vi "send_currentRamp-v02.vi"(0 "daq_ao":tag="Dev1/ao1", 1 "daq_ai":tag="Dev1/ai0:1", 5 "VoltageRampValuesCluster":T2, 7 "Sample Freq (Hz)":dbl min=0.0 max=40000.0, 9 "set holding (mV)":dbl, 13 "Number of Replicates":i16=1 min=1 max=10, 14 "error in":errorcluster) -> (4 "output cluster":T1, 6 "output waveform":waveform(dbl)[](graph), 8 "protocol response":waveform(dbl)[](graph) caption="jumptestMonitor", 10 "error out":errorcluster)   [LabVIEW 2019]
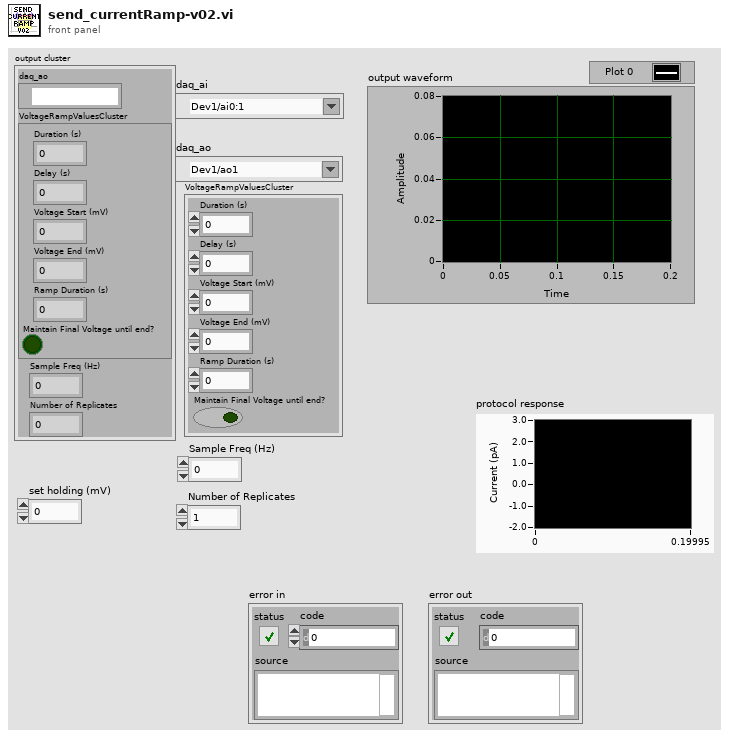
[diagram p1: front panel]
types:
  T1 = cluster{"daq_ao":tag, "VoltageRampValuesCluster":cluster{"Duration (s)":dbl, "Delay (s)":dbl, "Voltage Start (mV)":dbl, "Voltage End (mV)":dbl, "Ramp Duration (s)":dbl, "Maintain Final Voltage until end?":bool}, "Sample Freq (Hz)":dbl, "Number of Replicates":i16}
  T2 = cluster{"Duration (s)":dbl, "Delay (s)":dbl, "Voltage Start (mV)":dbl, "Voltage End (mV)":dbl, "Ramp Duration (s)":dbl, "Maintain Final Voltage until end?":bool}
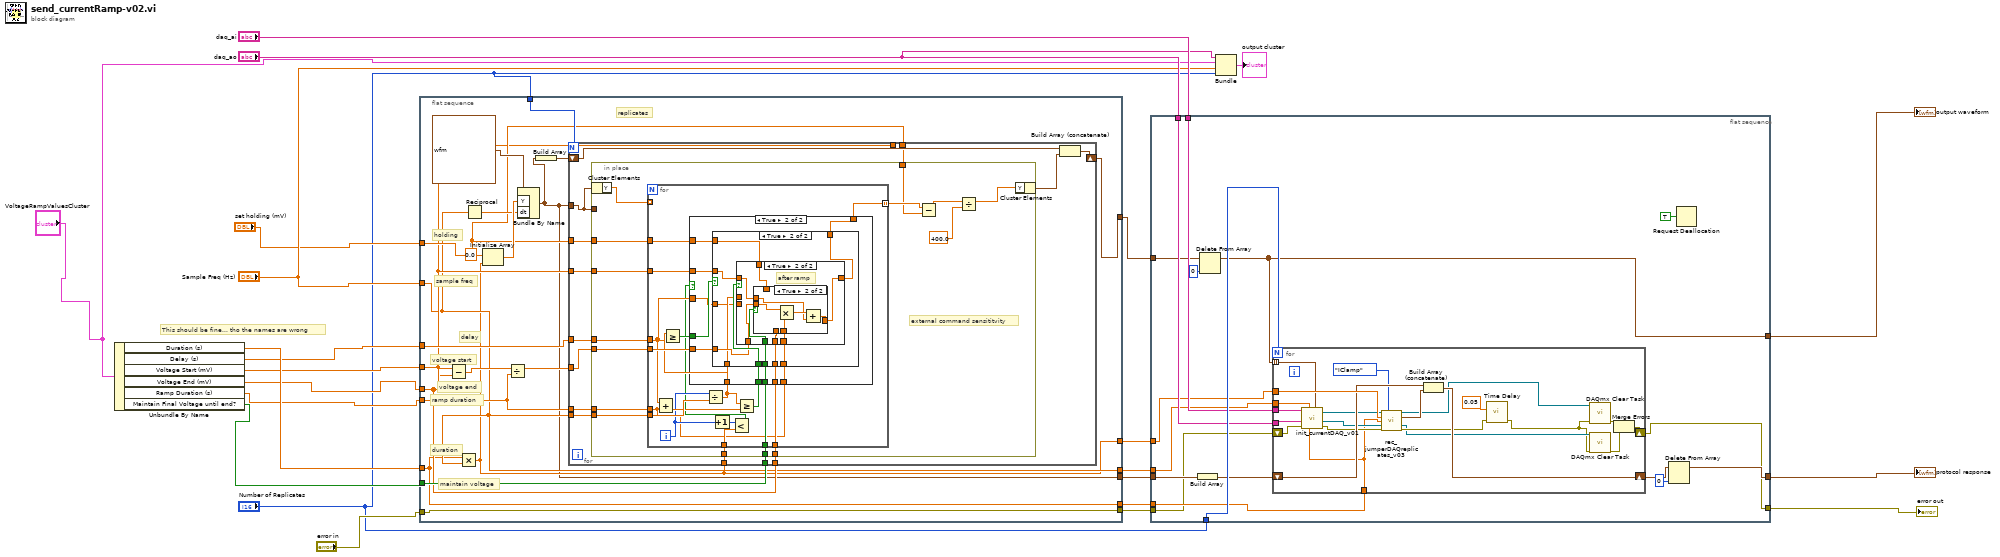
[diagram p0: block diagram]
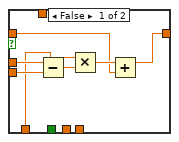
[diagram p4: hidden frame]
diagram:
  # "This should be fine... tho the names are wrong"
  n1 = Unbundle By Name("VoltageRampValuesCluster") -> ("Duration (s)"=w13:dbl, "Delay (s)"=w9:dbl, "Voltage Start (mV)"=w10:dbl, "Voltage End (mV)"=w11:dbl, "Ramp Duration (s)"=w12:dbl, "Maintain Final Voltage until end?"=w14:bool)
  n2 = flat-sequence {
    tunnel: w13 -> [w24]
    tunnel: "error in" -> [w33]
    tunnel: w9 -> [w38]
    tunnel: w10 -> [w28]
    tunnel: "Number of Replicates" -> [w43]
    tunnel: "Sample Freq (Hz)" -> [w27]
    tunnel: "set holding (mV)" -> [w30]
    tunnel: w11 -> [w31]
    tunnel: w12 -> [w37]
    tunnel: w14 -> [w35]
    tunnel: [w34] -> w5
    tunnel: [w28] -> _
    tunnel: [w33] -> w16
    tunnel: [w27] -> w4
    tunnel: [w26] -> w3
    tunnel: [w25] -> w2
    tunnel: [w24] -> w1
    frame #0 {
      # "maintain voltage"
      # "duration"
      # "ramp duration"
      # "voltage end"
      # "voltage start"
      # "delay"
      # "replicates"
      # "sample freq"
      # "holding"
      n3 = Subtract(x=w31, y=w28) -> (x-y=w32:dbl)
      n4 = Multiply(x=w24, y=w27) -> (x*y=w26:dbl)
      n5 = Reciprocal(x=w27) -> (1/x=w36:dbl)
      n6 = Initialize Array(0.0 ("element"), w26) -> (w40:dbl[])
      n7 = Divide(x=w32, y=w37) -> (x/y=w39:dbl)
      n8 = Bundle By Name(cluster=waveform(dbl) {"t0"=timestamp(0 s since 1904-01-01), "dt"=1.0, "Y"=[]} ("signal out"), "Y"=w40, "dt"=w36) -> (w25:waveform(dbl))
      n9 = Build Array(w25) -> (w42:waveform(dbl)[])
      n10 = for {
        N: w43 -> [_]
        shift-right: [w57] -> w34
        shift-left: w42 -> [w56]
        tunnel: w25 -> [w45]
        tunnel: w39 -> [w51]
        tunnel: w27 -> [w55]
        tunnel: w38 -> [w54]
        tunnel: w37 -> [w53]
        tunnel: w28 -> [w52]
        tunnel: w26 -> [w50]
        tunnel: w30 -> [w46]
        tunnel: w35 -> [w49]
        tunnel: w28 -> [_]
        tunnel: w30 -> [w48]
        tunnel: w31 -> [w47]
        n11 = in-place {
          in-place-border: w45 -> [_]
          in-place-border: w55 -> [w72]
          in-place-border: w54 -> [w71]
          in-place-border: w53 -> [w70]
          in-place-border: w52 -> [w69]
          in-place-border: w51 -> [w68]
          in-place-border: w50 -> [w67]
          in-place-border: w49 -> [w66]
          in-place-border: w48 -> [w65]
          in-place-border: w47 -> [w64]
          in-place-border: w46 -> [w61]
          # "external command sensititvity"
          n12 = in-place-cluster #1(w45) -> ("Y"=w59:dbl[])
          n13 = for {
            tunnel: [w73] -> w62 mode=indexing
            tunnel: w72 -> [w89]
            tunnel: w71 -> [w82]
            tunnel: w70 -> [w74]
            tunnel: w69 -> [w86]
            tunnel: w68 -> [w85]
            tunnel: w67 -> [w81]
            tunnel: w66 -> [w77]
            tunnel: w65 -> [w76]
            tunnel: w64 -> [w75]
            tunnel: w59 -> [_] mode=indexing
            i -> [w80]
            n14 = Add(x=w82, y=w74) -> (x+y=w83:dbl)
            n15 = Divide(x=w80, y=w89) -> (x/y=w84:dbl)
            n16 = Greater Or Equal?(x=w84, y=w82) -> (x >= y?=w88:bool)
            n17 = Increment(x=w80) -> (x+1=w78:i32)
            n18 = Less?(x=w78, y=w81) -> (x < y?=w79:bool)
            n19 = Greater Or Equal?(x=w84, y=w83) -> (x >= y?=w87:bool)
            n20 = case shown="True" w79 {
              tunnel: w88 -> [_ w101]
              tunnel: [w90 w100] -> w73
              tunnel: w87 -> [_ w99]
              tunnel: w86 -> [w90 w98]
              tunnel: w85 -> [_ w97]
              tunnel: w84 -> [_ w96]
              tunnel: w82 -> [_ w95]
              tunnel: w77 -> [_ w94]
              tunnel: w76 -> [_ w93]
              tunnel: w75 -> [_ w92]
              tunnel: w74 -> [_ w91]
              frame False {
                # "last sample"
              }
              frame True {
                n21 = case shown="True" w101 {
                  tunnel: [w102 w110] -> w100
                  tunnel: w99 -> [_ w112]
                  tunnel: w98 -> [w102 w111]
                  tunnel: w97 -> [_ w109]
                  tunnel: w96 -> [_ w108]
                  tunnel: w95 -> [_ w107]
                  tunnel: w94 -> [_ w106]
                  tunnel: w93 -> [_ w105]
                  tunnel: w92 -> [_ w104]
                  tunnel: w91 -> [_ w103]
                  frame False {
                    # "before delay"
                  }
                  frame True {
                    n22 = case shown="True" w112 {
                      tunnel: w111 -> [w113 w125]
                      tunnel: [w114 w124] -> w110
                      tunnel: w109 -> [w115 w121]
                      tunnel: w108 -> [w118 _]
                      tunnel: w107 -> [w119 _]
                      tunnel: w106 -> [_ w126]
                      tunnel: w105 -> [_ w123]
                      tunnel: w104 -> [_ w122]
                      tunnel: w103 -> [_ w120]
                      frame False {
                        n23 = Subtract(x=w118, y=w119) -> (x-y=w117:dbl)
                        n24 = Multiply(x=w115, y=w117) -> (x*y=w116:dbl)
                        n25 = Add(x=w116, y=w113) -> (x+y=w114:dbl)
                      }
                      frame True {
                        # "after ramp"
                        n26 = case shown="True" w126 {
                          tunnel: w125 -> [w127 w130]
                          tunnel: [w127 w131] -> w124
                          tunnel: w123 -> [_ _]
                          tunnel: w122 -> [_ _]
                          tunnel: w121 -> [_ w129]
                          tunnel: w120 -> [_ w128]
                          frame False {
                          }
                          frame True {
                            n27 = Multiply(x=w129, y=w128) -> (x*y=w132:dbl)
                            n28 = Add(x=w132, y=w130) -> (x+y=w131:dbl)
                          }
                        }
                      }
                    }
                  }
                }
              }
            }
          }
          n29 = Subtract(x=w62, y=w61) -> (x-y=w63:dbl[])
          n30 = Divide(x=w63, y=400.0) -> (x/y=w58:dbl[])
          n31 = in-place-cluster #1("Y"=w58) -> (w44:waveform(dbl))
        }
        n32 = Build Array (concatenate)(w56, w44) -> (w57:waveform(dbl)[])
      }
    }
  }
  n33 = flat-sequence {
    tunnel: [w141] -> w23
    tunnel: "daq_ai" -> [w144]
    tunnel: "daq_ao" -> [w143]
    tunnel: [w146] -> w20
    tunnel: "Number of Replicates" -> [w149]
    tunnel: [w135] -> w19
    tunnel: w16 -> [w134]
    tunnel: w5 -> [w140]
    tunnel: w4 -> [w139]
    tunnel: w3 -> [w138]
    tunnel: w2 -> [w137]
    tunnel: w1 -> [w136]
    frame #0 {
      n34 = Build Array(w137) -> (w148:waveform(dbl)[])
      n35 = Delete From Array(array=w140, index=0) -> (array with subset deleted=w141:waveform(dbl)[])  [unwired: 1 in, 1 out]
      n36 = for {
        N: w149 -> [_]
        tunnel: w138 -> [w171]
        shift-right: [w169] -> w147
        shift-left: w148 -> [w168]
        tunnel: w136 -> [w161]
        tunnel: w144 -> [w167]
        tunnel: w139 -> [w166]
        tunnel: w143 -> [w165]
        tunnel: w141 -> [w160] mode=indexing
        shift-right: [w152] -> w135
        shift-left: w134 -> [w151]
        n37 = call "init_currentDAQ_v01.vi"("protocol waveform"=w160, "Duration (s)"=w161, "Sample Freq (Hz)"=w166, "AO error in"=w151, "AO physical channels"=w165, "AI Physical Channel"=w167) -> ("AO error out"=w164:errorcluster, "AO task out"=w163:refnum<k21>, "AI task out"=w162:refnum<k21>)  [unwired: 1 in, 2 out]
        n38 = call "rec_jumperDAQreplicates_v03.vi"("AI task in"=w162, "which clamp"=enum16{"VClamp", "IClamp"}."IClamp", "number of samples"=w171, "Duration (s)"=w161, "AO task in"=w163, "error in"=w164) -> ("AI task out"=w156:refnum<k21>, "data out (pA or mV)"=w170:waveform(dbl), "AO task out"=w157:refnum<k21>, "error out"=w158:errorcluster)  [unwired: 6 in]
        n39 = Build Array (concatenate)(w168, w170) -> (w169:waveform(dbl)[])
        n40 = call "Time Delay"("error in (no error)"=w158, "Delay Time (s)"=0.05) -> ("error out"=w155:errorcluster)  [unwired: 9 in]
        n41 = call <vilib>:"DAQmx Clear Task.vi"("task in"=w156, "error in"=w155) -> ("error out"=w154:errorcluster)  [unwired: 13 in]
        n42 = call <vilib>:"DAQmx Clear Task.vi"("task in"=w157, "error in"=w155) -> ("error out"=w153:errorcluster)  [unwired: 13 in]
        n43 = Merge Errors(w154, w153) -> (w152:errorcluster)
      }
      n44 = Delete From Array(array=w147, index=0) -> (array with subset deleted=w146:waveform(dbl)[])  [unwired: 1 in, 1 out]
      n45 = Request Deallocation(TRUE ("flag")) -> ()
    }
  }
  n46 = Bundle("daq_ao"="daq_ao", "VoltageRampValuesCluster"="VoltageRampValuesCluster", "Sample Freq (Hz)"="Sample Freq (Hz)", "Number of Replicates"="Number of Replicates") -> (→"output cluster":T1)  [unwired: 1 in]
  "protocol response" <- w20
  "output waveform" <- w23
  "error out" <- w19
